vi "Load Threats.vi"(3 "errorIN":errorcluster, 5 "queryProjectileWt_Ref":refnum<vi>) -> (0 "error OUT":errorcluster, 2 "ProjectileWeights":string[](array[string]))   [LabVIEW 2010]
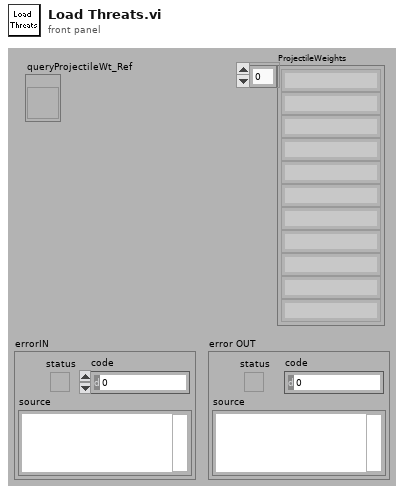
[diagram p1: front panel]
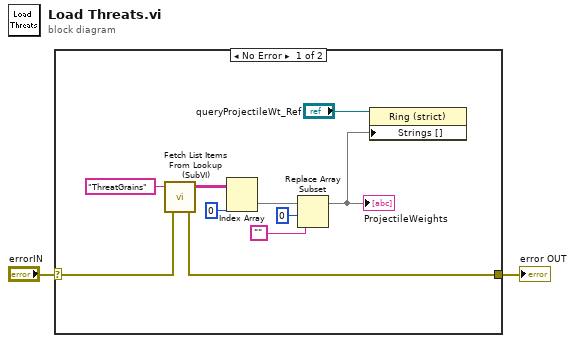
[diagram p0: block diagram]
diagram:
  n1 = case shown="No Error" "errorIN" {
    selector: "errorIN" -> [w8 w13]
    tunnel: [w7 w13] -> w1
    frame No Error {
      n2 = call "Fetch List Items From Lookup (SubVI).vi"("error IN"=w8, "Query"="ThreatGrains" ("lookup table name")) -> ("error OUT"=w7:errorcluster, "recordset data"=w12:string[][])  [unwired: 2 out]
      n3 = Index Array(array=w12, index (col)=0 ("disabled index (col)")) -> (element=w3:string[])  [unwired: 1 in]
      n4 = Replace Array Subset(array=w3, new element="" ("new element/subarray"), index=0) -> (w4:string[])
      "ProjectileWeights" <- w4
      n5 = property class="Ring (strict)"(reference="queryProjectileWt_Ref", "Strings []"=w4) -> ()  [unwired: 1 in, 2 out]
    }
    frame Error {
    }
  }
  "error OUT" <- w1
